vi "Periodic Tasks.vi"(8 "error in":errorcluster) -> ()   [LabVIEW 2013]
doc: "This VI runs in parallel to other tasks. It can contain as many user-defined periodic loops as you need. These can carry out PID or other sorts of timed response."
uses:
  <vilib>/Rock Robotics/SystemInterfaces/Utilities/FPGA_UtilitiesLED Source.ctl
  <vilib>/Rock Robotics/SystemInterfaces/Utilities/FPGA_UtilitiesLED State.ctl
  <vilib>/Rock Robotics/WPI/Relay/WPI_RelayValue.ctl
  <vilib>/Rock Robotics/WPI/Ultrasonic/WPI_UltrasonicRangeUnits.ctl
  Robot Global Data.vi
  Device Refrences.vi
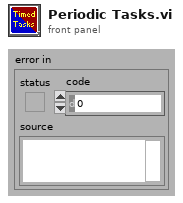
[diagram p1: front panel]
types:
  T1 = typedef "WPI_SolenoidValue.ctl" = enum16{"Off", "On", "Forward", "Reverse"}
  T2 = cluster{"Drive Output Values":dbl[], "Shooter Solenoid":T1, "Pickup Solenoid":T1, "Pickup Motor":dbl, "Ejecter Solenoid":T1}
  T3 = typedef "WPI_JoystickButtonState.ctl" = cluster{"Button 1":bool, "Button 2":bool, "Button 3":bool, "Button 4":bool, "Button 5":bool, "Button 6":bool, "Button 7":bool, "Button 8":bool, "Button 9":bool, "Button 10":bool, "Button 11":bool, "Button 12":bool}
  T4 = cluster{"Axes":cluster{"axis 1 (x)":dbl, "axis 2 (y)":dbl, "axis 3 (throttle)":dbl, "axis 4":dbl, "axis 5":dbl, "axis 6":dbl}, "Buttons":T3}
  T5 = cluster{"Compressor running":bool, "Compressor enabled":bool, "Right Encoder":dbl, "Left Encoder":dbl, "Ultrasonic Sensor":dbl, "Light Sensor":dbl, "Gyro":dbl}
  T6 = cluster{"axis 1 (x)":dbl, "axis 2 (y)":dbl, "axis 3 (throttle)":dbl, "axis 4":dbl, "axis 5":dbl, "axis 6":dbl}
  T7 = cluster{"Distance from tape":dbl, "1st Shoot Distance":dbl, "2nd Shoot Distance":dbl, "Auto Routine":dbl, "Start Position":dbl}
  T8 = typedef "WPI_JoystickDevRef.ctl" = cluster{"Device":T9}
  T9 = typedef "WPI_JoystickDeviceEnum.ctl" = enum16{"USB 1", "USB 2", "USB 3", "USB 4", "Kinect 1", "Kinect 2"}
  T10 = enum16{"1 3-axis Joystick", "2 2-axis Joysticks"}
  T11 = cluster{"Drive Y":dbl, "Drive X":dbl, "Extend Pickup":bool, "Retract Pickup":bool, "Shoot Ball":bool, "Short Range":bool, "Eject Ball":bool, "Pickup Motor":dbl, "Long Range":bool, "Retract Shooter":bool, "Speed Throttle":bool, "Specified Range":bool}
  T12 = enum16{"Simulator Robot", "Alpinista", "2014 Robot"}
  T13 = typedef "WPI_CompressorDevRef.ctl" = cluster{"DevStatus":errorcluster, "DigitalInputDevRef":T14, "RelayDevRef":T17}
  T14 = typedef "WPI_DigitalInputDevRef.ctl" = cluster{"DevStatus":errorcluster, "DIO Channel":T15, "Digital Module":T16}
  T15 = typedef "FPGA_DIOChannel.ctl" = enum8{"DIO 1", "DIO 2", "DIO 3", "DIO 4", "DIO 5", "DIO 6", "DIO 7", "DIO 8", "DIO 9", "DIO 10", "DIO 11", "DIO 12", "DIO 13", "DIO 14", "Invalid"}
  T16 = typedef "FPGA_TypedefDigitalModule.ctl" = enum16{"Digital Module 1", "Digital Module 2"}
  T17 = typedef "WPI_RelayDevRef.ctl" = cluster{"DevStatus":errorcluster, "Relay Channel":T18, "Digital Module":T16, "Relay Direction":T19}
  T18 = typedef "FPGA_DIORelayChannel.ctl" = enum8{"Relay 1", "Relay 2", "Relay 3", "Relay 4", "Relay 5", "Relay 6", "Relay 7", "Relay 8", "Invalid"}
  T19 = typedef "WPI_RelayDirection.ctl" = enum16{"Both directions", "Forward only", "Reverse only"}
  T20 = typedef "FPGA_UtilitiesLED State.ctl" = enum16{"Off", "On", "Toggle"}
  T21 = typedef "FPGA_UtilitiesLED Source.ctl" = enum16{"User LED", "FPGA LED"}
  T22 = typedef "WPI_RelayValue.ctl" = enum16{"Off", "On", "Forward", "Reverse"}
  T23 = typedef "WPI_UltrasonicRangeUnits.ctl" = enum16{"inches", "mm"}
  T24 = typedef "WPI_GyroDevRef.ctl" = cluster{"DevStatus":errorcluster, "Analog Module":T25, "Analog Channel":T26, "Offset":dbl, "Gain (VoltsPerDegree/Second)":dbl}
  T25 = typedef "FPGA_TypedefAnalogModule.ctl" = enum16{"Analog Module 1", "Analog Module 2"}
  T26 = typedef "FPGA_AIChannel.ctl" = enum8{"AI 1", "AI 2", "AI 3", "AI 4", "AI 5", "AI 6", "AI 7", "AI 8", "Invalid"}
  T27 = typedef "WPI_UltrasonicDeviceRef.ctl" = cluster{"DevStatus":errorcluster, "Ping Digital Module":T16, "Echo Digital Module":T16, "Ping Channel":T15, "Echo Channel":T15, "CntIndex":T28}
  T28 = typedef "FPGA_CounterCtrSystemIndex.ctl" = enum8{"Ctr 0", "Ctr 1", "Ctr 2", "Ctr 3", "Ctr 4", "Ctr 5", "Ctr 6", "Ctr 7", "Invalid"}
  T29 = typedef "WPI_CounterDevRef.ctl" = cluster{"DevStatus":errorcluster, "CntIndex":T28}
  T30 = typedef "WPI_AnalogChannelDevRef.ctl" = cluster{"DevStatus":errorcluster, "Analog Module":T25, "Analog Channel":T26}
  T31 = typedef "WPI_EncoderDevRef.ctl" = cluster{"DevStatus":errorcluster, "EncoderIndex":T32, "CounterIndex":T28, "DistancePerCount":dbl, "Decoding Type":T33}
  T32 = typedef "FPGA_EncoderIdx.ctl" = enum8{"Enc 0", "Enc 1", "Enc 2", "Enc 3", "Invalid"}
  T33 = typedef "WPI_EncoderType.ctl" = enum16{"1x", "2x", "4x"}
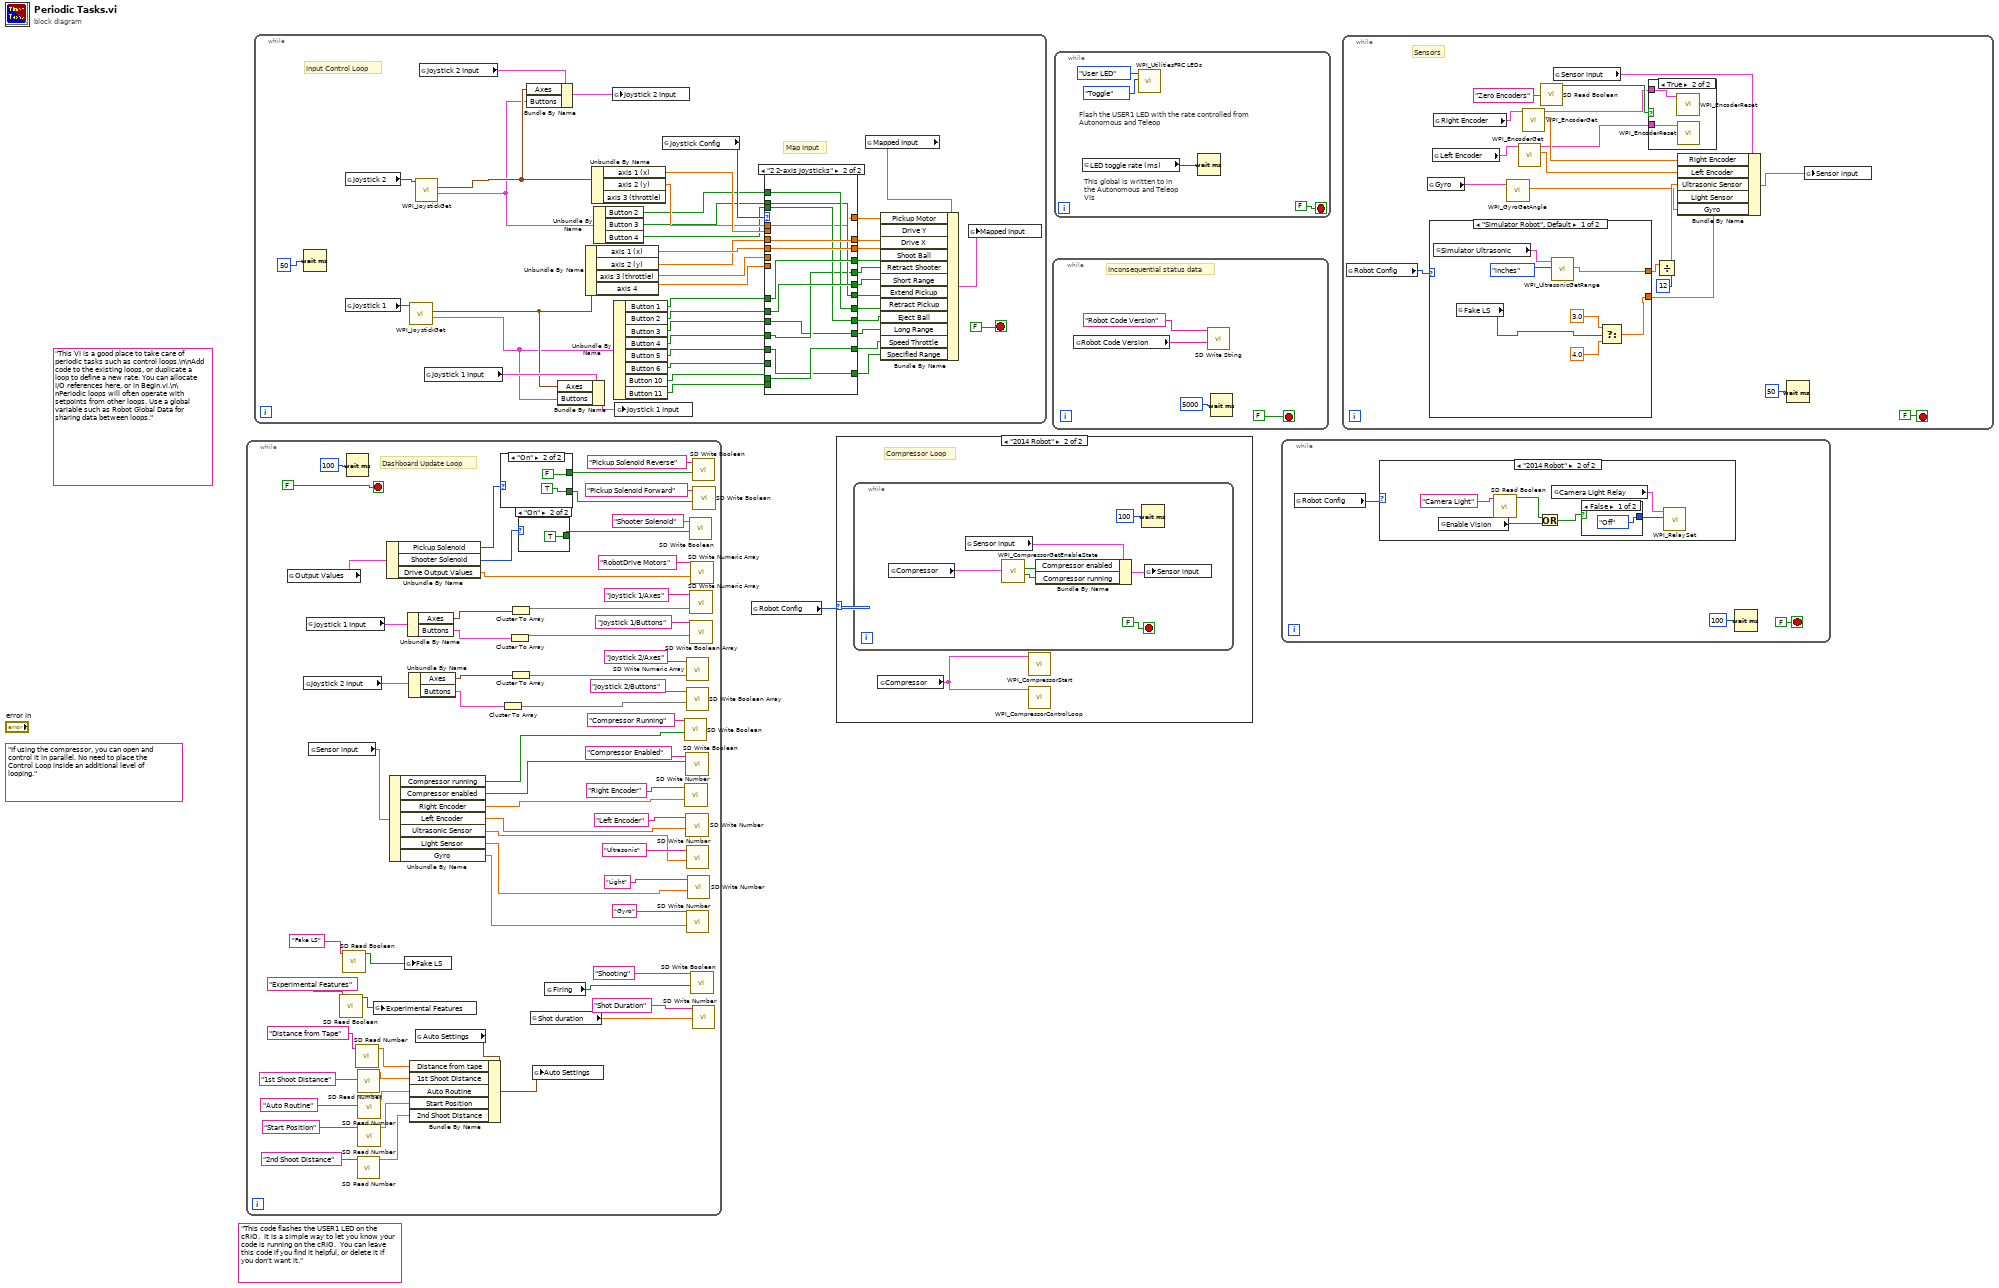
[diagram p0: block diagram]
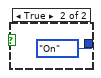
[diagram p3: hidden frame]
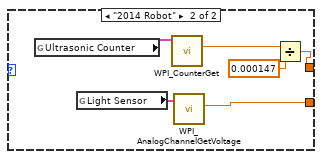
[diagram p5: hidden frame]
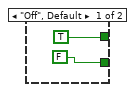
[diagram p7: hidden frame]
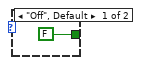
[diagram p8: hidden frame]
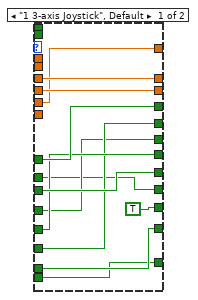
[diagram p9: hidden frame]
diagram:
  (unwired) "If using the compressor, you can open and control it in parallel. No need to place the Control Loop inside an additional level of looping."
  (unwired) "This code flashes the USER1 LED on the cRIO.  It is a simple way to let you know your code is running on the cRIO.  You can leave this code if you find it helpful, or delete it if you don't want it."
  (unwired) "This VI is a good place to take care of periodic tasks such as control loops.\n\nAdd code to the existing loops, or duplicate a loop to define a new rate. You can allocate I/O references here, or in Begin.vi.\n\nPeriodic loops will often operate with setpoints from other loops. Use a global variable such as Robot Global Data for sharing data between loops."
  n1 = while {
    stop <- FALSE stop-if-true
    # "Dashboard Update Loop"
    n2 = global read "Robot Global Data.vi" "Output Values"() -> (w41:T2)
    n3 = global read "Robot Global Data.vi" "Joystick 2 Input"() -> (w54:T4)
    n4 = global read "Robot Global Data.vi" "Joystick 1 Input"() -> (w57:T4)
    n5 = global read "Robot Global Data.vi" "Sensor input"() -> (w46:T5)
    n6 = call <vilib>:"SD Read Boolean.vi"("Name"="Experimental Features") -> ("Boolean"=w9:bool)  [unwired: 8 in, 2 out]
    n7 = call <vilib>:"SD Read Boolean.vi"("Name"="Fake LS") -> ("Boolean"=w22:bool)  [unwired: 8 in, 2 out]
    n8 = Wait (ms)(milliseconds to wait=u32 100) -> ()  [unwired: 1 out]
    n9 = call <vilib>:"SD Read Number.vi"("Name"="Distance from Tape") -> ("Numeric"=w13:dbl)  [unwired: 8 in, 2 out]
    n10 = call <vilib>:"SD Read Number.vi"("Name"="1st Shoot Distance") -> ("Numeric"=w12:dbl)  [unwired: 8 in, 2 out]
    n11 = call <vilib>:"SD Read Number.vi"("Name"="2nd Shoot Distance") -> ("Numeric"=w2:dbl)  [unwired: 8 in, 2 out]
    n12 = call <vilib>:"SD Read Number.vi"("Name"="Auto Routine") -> ("Numeric"=w10:dbl)  [unwired: 8 in, 2 out]
    n13 = call <vilib>:"SD Read Number.vi"("Name"="Start Position") -> ("Numeric"=w6:dbl)  [unwired: 8 in, 2 out]
    n14 = global write "Robot Global Data.vi" "Experimental Features"(w9) -> ()
    n15 = Unbundle By Name(w41) -> ("Pickup Solenoid"=w37:T1, "Shooter Solenoid"=w34:T1, "Drive Output Values"=w40:dbl[])
    n16 = Unbundle By Name(w46) -> ("Compressor running"=w44:bool, "Compressor enabled"=w45:bool, "Right Encoder"=w29:dbl, "Left Encoder"=w30:dbl, "Ultrasonic Sensor"=w26:dbl, "Light Sensor"=w25:dbl, "Gyro"=w5:dbl)
    n17 = global write "Robot Global Data.vi" "Fake LS"(w22) -> ()
    n18 = Unbundle By Name(w57) -> ("Axes"=w56:T6, "Buttons"=w55:T3)
    n19 = Unbundle By Name(w54) -> ("Axes"=w49:T6, "Buttons"=w48:T3)
    n20 = global read "Robot Global Data.vi" "Auto Settings"() -> (w17:T7)
    n21 = Bundle By Name(cluster=w17, "Distance from tape"=w13, "1st Shoot Distance"=w12, "Auto Routine"=w10, "Start Position"=w6, "2nd Shoot Distance"=w2) -> (w16:T7)
    n22 = case shown="\"On\"" w37 {
      tunnel: [TRUE FALSE] -> w33
      tunnel: [FALSE TRUE] -> w32
      frame "Off", Default {
      }
      frame "On" {
      }
    }
    n23 = Cluster To Array(cluster=w48) -> (array=w53:bool[])
    n24 = Cluster To Array(cluster=w55) -> (array=w58:bool[])
    n25 = Cluster To Array(cluster=w56) -> (array=w60:dbl[])
    n26 = Cluster To Array(cluster=w49) -> (array=w51:dbl[])
    n27 = case shown="\"On\"" w34 {
      tunnel: [FALSE TRUE] -> w38
      frame "Off", Default {
      }
      frame "On" {
      }
    }
    n28 = global read "Robot Global Data.vi" "Shot duration"() -> (w20:dbl)
    n29 = global write "Robot Global Data.vi" "Auto Settings"(w16) -> ()
    n30 = global read "Robot Global Data.vi" "Firing"() -> (w19:bool)
    n31 = call <vilib>:"SD Write Boolean.vi"("Boolean"=w44, "Name"="Compressor Running") -> ()  [unwired: 8 in, 2 out]
    n32 = call <vilib>:"SD Write Number.vi"("Numeric"=w29, "Name"="Right Encoder") -> ()  [unwired: 8 in, 2 out]
    n33 = call <vilib>:"SD Write Boolean.vi"("Boolean"=w45, "Name"="Compressor Enabled") -> ()  [unwired: 8 in, 2 out]
    n34 = call <vilib>:"SD Write Number.vi"("Numeric"=w30, "Name"="Left Encoder") -> ()  [unwired: 8 in, 2 out]
    n35 = call <vilib>:"SD Write Numeric Array.vi"("Numeric Array"=w51, "Name"="Joystick 2/Axes") -> ()  [unwired: 8 in, 2 out]
    n36 = call <vilib>:"SD Write Boolean Array.vi"("Boolean Array"=w53, "Name"="Joystick 2/Buttons") -> ()  [unwired: 8 in, 2 out]
    n37 = call <vilib>:"SD Write Number.vi"("Numeric"=w26, "Name"="Ultrasonic") -> ()  [unwired: 8 in, 2 out]
    n38 = call <vilib>:"SD Write Number.vi"("Numeric"=w5, "Name"="Gyro") -> ()  [unwired: 8 in, 2 out]
    n39 = call <vilib>:"SD Write Number.vi"("Numeric"=w25, "Name"="Light") -> ()  [unwired: 8 in, 2 out]
    n40 = call <vilib>:"SD Write Boolean.vi"("Boolean"=w38, "Name"="Shooter Solenoid") -> ()  [unwired: 8 in, 2 out]
    n41 = call <vilib>:"SD Write Numeric Array.vi"("Numeric Array"=w60, "Name"="Joystick 1/Axes") -> ()  [unwired: 8 in, 2 out]
    n42 = call <vilib>:"SD Write Boolean Array.vi"("Boolean Array"=w58, "Name"="Joystick 1/Buttons") -> ()  [unwired: 8 in, 2 out]
    n43 = call <vilib>:"SD Write Numeric Array.vi"("Numeric Array"=w40, "Name"="RobotDrive Motors") -> ()  [unwired: 8 in, 2 out]
    n44 = call <vilib>:"SD Write Boolean.vi"("Boolean"=w19, "Name"="Shooting") -> ()  [unwired: 8 in, 2 out]
    n45 = call <vilib>:"SD Write Boolean.vi"("Boolean"=w33, "Name"="Pickup Solenoid Reverse") -> ()  [unwired: 8 in, 2 out]
    n46 = call <vilib>:"SD Write Number.vi"("Numeric"=w20, "Name"="Shot Duration") -> ()  [unwired: 8 in, 2 out]
    n47 = call <vilib>:"SD Write Boolean.vi"("Boolean"=w32, "Name"="Pickup Solenoid Forward") -> ()  [unwired: 8 in, 2 out]
  }
  n48 = while {
    stop <- FALSE stop-if-true
    # "Input Control Loop"
    # "Map Input"
    n49 = Wait (ms)(milliseconds to wait=u32 50) -> ()  [unwired: 1 out]
    n50 = global read "Device Refrences.vi" "Joystick 2"() -> (w92:T8)
    n51 = global read "Device Refrences.vi" "Joystick 1"() -> (w111:T8)
    n52 = call <vilib>:"WPI_JoystickGet.vi"("JoystickDevRef"=w111) -> ("Buttons"=w97:T3, "Axes"=w98:T6)  [unwired: 4 in, 1 out]
    n53 = call <vilib>:"WPI_JoystickGet.vi"("JoystickDevRef"=w92) -> ("Buttons"=w93:T3, "Axes"=w94:T6)  [unwired: 4 in, 1 out]
    n54 = global read "Robot Global Data.vi" "Joystick 2 Input"() -> (w95:T4)
    n55 = global read "Robot Global Data.vi" "Joystick 1 Input"() -> (w100:T4)
    n56 = Bundle By Name(cluster=w95, "Axes"=w94, "Buttons"=w93) -> (w96:T4)
    n57 = Bundle By Name(cluster=w100, "Axes"=w98, "Buttons"=w97) -> (w99:T4)
    n58 = Unbundle By Name(w98) -> ("axis 1 (x)"=w109:dbl, "axis 2 (y)"=w108:dbl, "axis 3 (throttle)"=w107:dbl, "axis 4"=w102:dbl)
    n59 = Unbundle By Name(w94) -> ("axis 1 (x)"=w101:dbl, "axis 2 (y)"=w91:dbl)  [unwired: 1 out]
    n60 = Unbundle By Name(w93) -> ("Button 2"=w81:bool, "Button 3"=w80:bool, "Button 4"=w76:bool)
    n61 = global write "Robot Global Data.vi" "Joystick 2 Input"(w96) -> ()
    n62 = Unbundle By Name(w97) -> ("Button 1"=w90:bool, "Button 2"=w89:bool, "Button 3"=w88:bool, "Button 4"=w84:bool, "Button 5"=w83:bool, "Button 6"=w82:bool, "Button 10"=w72:bool, "Button 11"=w70:bool)
    n63 = global write "Robot Global Data.vi" "Joystick 1 Input"(w99) -> ()
    n64 = global read "Robot Global Data.vi" "Joystick Config"() -> (w110:T10)
    n65 = case shown="\"2 2-axis Joysticks\"" w110 {
      tunnel: w109 -> [w125 w137]
      tunnel: w108 -> [w124 w136]
      tunnel: w107 -> [w117 _]
      tunnel: [w125 w137] -> w104
      tunnel: [w124 w136] -> w103
      tunnel: w102 -> [_ _]
      tunnel: w101 -> [_ _]
      tunnel: w91 -> [_ w130]
      tunnel: w90 -> [w123 w135]
      tunnel: w89 -> [w118 w134]
      tunnel: w88 -> [w122 w127]
      tunnel: [w122 w133] -> w86
      tunnel: [w123 w135] -> w87
      tunnel: [w121 w132] -> w85
      tunnel: w84 -> [w119 w129]
      tunnel: w83 -> [w121 w126]
      tunnel: w82 -> [w120 _]
      tunnel: w81 -> [_ w133]
      tunnel: w80 -> [_ w132]
      tunnel: [w120 w129] -> w79
      tunnel: [w119 w134] -> w78
      tunnel: [w118 w131] -> w77
      tunnel: w76 -> [_ w131]
      tunnel: [w117 w130] -> w75
      tunnel: [TRUE w127] -> w74
      tunnel: [w115 w128] -> w73
      tunnel: w72 -> [w115 w128]
      tunnel: [w114 w126] -> w71
      tunnel: w70 -> [w114 _]
      frame "1 3-axis Joystick", Default {
      }
      frame "2 2-axis Joysticks" {
      }
    }
    n66 = global read "Robot Global Data.vi" "Mapped Input"() -> (w105:T11)
    n67 = Bundle By Name(cluster=w105, "Pickup Motor"=w75, "Drive Y"=w103, "Drive X"=w104, "Shoot Ball"=w87, "Retract Shooter"=w79, "Short Range"=w78, "Extend Pickup"=w85, "Retract Pickup"=w86, "Eject Ball"=w77, "Long Range"=w74, "Speed Throttle"=w73, "Specified Range"=w71) -> (w106:T11)
    n68 = global write "Robot Global Data.vi" "Mapped Input"(w106) -> ()
  }
  n69 = global read "Robot Global Data.vi" "Robot Config"() -> (w1:T12)
  n70 = case shown="\"2014 Robot\"" w1 {
    frame "Simulator Robot", Default {
    }
    frame "2014 Robot" {
      # "Compressor Loop"
      n71 = while {
        stop <- FALSE stop-if-true
        n72 = global read "Device Refrences.vi" "Compressor"() -> (w145:T13)
        n73 = global read "Robot Global Data.vi" "Sensor input"() -> (w144:T5)
        n74 = call <vilib>:"WPI_CompressorGetEnableState.vi"("CompressorDevRef"=w145) -> ("Compressor Running"=w139:bool, "Enabled"=w140:bool)  [unwired: 7 in, 2 out]
        n75 = Bundle By Name(cluster=w144, "Compressor enabled"=w140, "Compressor running"=w139) -> (w143:T5)
        n76 = Wait (ms)(milliseconds to wait=u32 100) -> ()  [unwired: 1 out]
        n77 = global write "Robot Global Data.vi" "Sensor input"(w143) -> ()
      }
      n78 = global read "Device Refrences.vi" "Compressor"() -> (w138:T13)
      n79 = call <vilib>:"WPI_CompressorStart.vi"("CompressorDevRef"=w138) -> ()  [unwired: 1 in, 10 out]
      n80 = call <vilib>:"WPI_CompressorControlLoop.vi"("CompressorDevRef"=w138) -> ()  [unwired: 11 in]
    }
  }
  n81 = while {
    stop <- FALSE stop-if-true
    # "Inconsequential status data"
    n82 = global read "Robot Global Data.vi" "Robot Code Version"() -> (w146:string)
    n83 = call <vilib>:"SD Write String.vi"("String"=w146, "Name"="Robot Code Version") -> ()  [unwired: 8 in, 2 out]
    n84 = Wait (ms)(milliseconds to wait=u32 5000) -> ()  [unwired: 1 out]
  }
  n85 = while {
    stop <- FALSE stop-if-true
    # "This global is written to in the Autonomous and Teleop VIs"
    # "Flash the USER1 LED with the rate controlled from Autonomous and Teleop"
    n86 = global read "Robot Global Data.vi" "LED toggle rate (ms)"() -> (w150:u32)
    n87 = call <vilib>:"WPI_UtilitiesFRC LEDs.vi"("State"=FPGA_UtilitiesLED_State."Toggle", "LED Type"=FPGA_UtilitiesLED_Source."User LED") -> ()  [unwired: 1 in, 9 out]
    n88 = Wait (ms)(milliseconds to wait=w150) -> ()  [unwired: 1 out]
  }
  n89 = while {
    stop <- FALSE stop-if-true
    n90 = global read "Robot Global Data.vi" "Robot Config"() -> (w154:T12)
    n91 = case shown="\"2014 Robot\"" w154 {
      frame "Simulator Robot", Default {
      }
      frame "2014 Robot" {
        n92 = global read "Robot Global Data.vi" "Enable Vision"() -> (w157:bool)
        n93 = call <vilib>:"SD Read Boolean.vi"("Name"="Camera Light") -> ("Boolean"=w158:bool)  [unwired: 8 in, 2 out]
        n94 = Or(x=w158, y=w157) -> (x .or. y?=w159:bool)
        n95 = global read "Device Refrences.vi" "Camera Light Relay"() -> (w162:T17)
        n96 = case shown="False" w159 {
          tunnel: [WPI_RelayValue."Off" ("RelayValue") WPI_RelayValue."On" ("RelayValue")] -> w161
          frame False {
          }
          frame True {
          }
        }
        n97 = call <vilib>:"WPI_RelaySet.vi"("RelayValue"=w161, "RelayDevRef"=w162) -> ()  [unwired: 8 in, 2 out]
      }
    }
    n98 = Wait (ms)(milliseconds to wait=u32 100) -> ()  [unwired: 1 out]
  }
  n99 = while {
    stop <- FALSE stop-if-true
    # "Sensors"
    n100 = global read "Robot Global Data.vi" "Robot Config"() -> (w176:T12)
    n101 = global read "Device Refrences.vi" "Gyro"() -> (w165:T24)
    n102 = case shown="\"Simulator Robot\", Default" w176 {
      tunnel: [w190 w196] -> w168
      tunnel: [w188 w193] -> w175
      frame "Simulator Robot", Default {
        n103 = global read "Device Refrences.vi" "Simulator Ultrasonic"() -> (w192:T27)
        n104 = global read "Robot Global Data.vi" "Fake LS"() -> (w186:bool)
        n105 = call <vilib>:"WPI_UltrasonicGetRange.vi"("Range Units"=WPI_UltrasonicRangeUnits."inches", "UltrasonicDevRef"=w192) -> ("Distance"=w190:dbl)  [unwired: 7 in, 2 out]
        n106 = Select(t=3.0, s=w186, f=4.0) -> (s? t:f=w188:dbl)
      }
      frame "2014 Robot" {
        n107 = global read "Device Refrences.vi" "Ultrasonic Counter"() -> (w197:T29)
        n108 = global read "Device Refrences.vi" "Light Sensor"() -> (w194:T30)
        n109 = call <vilib>:"WPI_CounterGet.vi"("CounterDevRef in"=w197) -> ("Period (sec)"=w195:dbl)  [unwired: 5 in, 5 out]
        n110 = call <vilib>:"WPI_AnalogChannelGetVoltage.vi"("AIDeviceRef"=w194) -> ("Voltage"=w193:dbl)  [unwired: 8 in, 2 out]
        n111 = Divide(x=w195, y=0.000147) -> (x/y=w196:dbl)
      }
    }
    n112 = global read "Device Refrences.vi" "Left Encoder"() -> (w180:T31)
    n113 = global read "Device Refrences.vi" "Right Encoder"() -> (w182:T31)
    n114 = call <vilib>:"WPI_GyroGetAngle.vi"("GyroDevRef"=w165) -> ("Angle"=w166:dbl)  [unwired: 7 in, 3 out]
    n115 = call <vilib>:"WPI_EncoderGet.vi"("EncoderDevRef"=w180) -> ("Distance"=w179:dbl, "EncoderDevRef"=w172:T31)  [unwired: 5 in, 4 out]
    n116 = call <vilib>:"WPI_EncoderGet.vi"("EncoderDevRef"=w182) -> ("Distance"=w178:dbl, "EncoderDevRef"=w171:T31)  [unwired: 5 in, 4 out]
    n117 = call <vilib>:"SD Read Boolean.vi"("Name"="Zero Encoders") -> ("Boolean"=w173:bool)  [unwired: 8 in, 2 out]
    n118 = global read "Robot Global Data.vi" "Sensor input"() -> (w181:T5)
    n119 = case shown="True" w173 {
      tunnel: w172 -> [_ w185]
      tunnel: w171 -> [_ w184]
      frame False {
      }
      frame True {
        n120 = call <vilib>:"WPI_EncoderReset.vi"("EncoderDevRef"=w184) -> ()  [unwired: 9 in, 2 out]
        n121 = call <vilib>:"WPI_EncoderReset.vi"("EncoderDevRef"=w185) -> ()  [unwired: 9 in, 2 out]
      }
    }
    n122 = Divide(x=w168, y=12) -> (x/y=w167:dbl)
    n123 = Bundle By Name(cluster=w181, "Right Encoder"=w178, "Left Encoder"=w179, "Ultrasonic Sensor"=w167, "Light Sensor"=w175, "Gyro"=w166) -> (w170:T5)
    n124 = Wait (ms)(milliseconds to wait=u32 50) -> ()  [unwired: 1 out]
    n125 = global write "Robot Global Data.vi" "Sensor input"(w170) -> ()
  }
